vi "TEST-JSON-RPC.vi"() -> ()   [LabVIEW 2019, in "JSON-RPC.lvclass"]
uses:
  JSON-RPC.lvclass
  typedefs/Request--Cluster.ctl
  <vilib>/numeric/Random Number (Range) DBL.vi
  2af6048a-36b0-468c-b9d5-439df6bbc06a.vi
  423c0946-e876-4033-917c-c4e0f5a656b4.vi
  ba7f8204-1185-4351-9b6f-00361c30192e.vi
  2af6048a-36b0-468c-b9d5-439df6bbc06a.vi/56c0d29a-bd12-4556-9f6c-07d4d8114690.vi
  lv-venv/lv.lib/vi.lib/JDP Science/JSONtext/Make JSON Array.vi
  API/Create Batch Response.vi/8dac1c84-94f0-4a52-a653-2d1a946a353f.vi
  private/Parse Response-JSONtext.vi
  2af6048a-36b0-468c-b9d5-439df6bbc06a.vi/56c0d29a-bd12-4556-9f6c-07d4d8114690.vi/b1ff17d3-7a39-46cb-8eb5-aa197442e16a.vi
  API/Create Batch Response.vi/8dac1c84-94f0-4a52-a653-2d1a946a353f.vi/080af00f-872a-404d-81fb-91aec086d127.vi
  private/Parse Response-JSONtext.vi/7ce7fba8-9f44-478d-b6cb-b571ff29f2f5.vi
  private/Parse Response-JSONtext.vi/8c905beb-ab4c-49e3-b5c6-2c663b7b30d7.vi
  private/Parse Response-JSONtext.vi/fce5892e-0c40-47e1-88e0-6c122aadefe2.vi
  2af6048a-36b0-468c-b9d5-439df6bbc06a.vi/56c0d29a-bd12-4556-9f6c-07d4d8114690.vi/b1ff17d3-7a39-46cb-8eb5-aa197442e16a.vi/28d9b5f0-560b-4ba5-abe5-6e3ff87b2b6b.vi
  2af6048a-36b0-468c-b9d5-439df6bbc06a.vi/56c0d29a-bd12-4556-9f6c-07d4d8114690.vi/b1ff17d3-7a39-46cb-8eb5-aa197442e16a.vi/0d2768a8-5a07-4864-b3c8-f491049a930f.vi
  2af6048a-36b0-468c-b9d5-439df6bbc06a.vi/56c0d29a-bd12-4556-9f6c-07d4d8114690.vi/b1ff17d3-7a39-46cb-8eb5-aa197442e16a.vi/1e98635b-27c0-4b27-a2b5-38e38c963eb7.vi
  2af6048a-36b0-468c-b9d5-439df6bbc06a.vi/56c0d29a-bd12-4556-9f6c-07d4d8114690.vi/b1ff17d3-7a39-46cb-8eb5-aa197442e16a.vi/0d772b24-2de1-48ba-989a-96e16cd43241.vi
  2af6048a-36b0-468c-b9d5-439df6bbc06a.vi/56c0d29a-bd12-4556-9f6c-07d4d8114690.vi/b1ff17d3-7a39-46cb-8eb5-aa197442e16a.vi/3a44731f-0131-47ed-b9ac-c843c255cdb0.vi
  API/Create Batch Response.vi/8dac1c84-94f0-4a52-a653-2d1a946a353f.vi/080af00f-872a-404d-81fb-91aec086d127.vi/ddd97ab0-f880-4d62-a12b-adbfa2b80abd.vi
  API/Create Batch Response.vi/8dac1c84-94f0-4a52-a653-2d1a946a353f.vi/080af00f-872a-404d-81fb-91aec086d127.vi/db6e2d89-34ae-420f-86ba-38671ee62ba9.vi
  API/Create Batch Response.vi/8dac1c84-94f0-4a52-a653-2d1a946a353f.vi/080af00f-872a-404d-81fb-91aec086d127.vi/9674d577-b062-4377-a879-970cb02c3975.vi
  private/Create Error Object.vi
  lv-venv/lv.lib/vi.lib/JDP Science/JSONtext/Find Item.vi
  lv-venv/lv.lib/vi.lib/JDP Science/JSONtext/String Subset.vi
  <vilib>/Utility/Data Type/Get Type Information.vi
  lv-venv/lv.lib/vi.lib/JDP Science/JSONtext/Variant to JSON Text.vi
  lv-venv/lv.lib/vi.lib/JDP Science/JSONtext/Set Item.vi
  private/Create ID.vi
  lv-venv/lv.lib/vi.lib/JDP Science/JSONtext/support/Format JSON Array Text.vi
  lv-venv/lv.lib/vi.lib/JDP Science/JSONtext/JSON text to Variant.vi
  lv-venv/lv.lib/vi.lib/JDP Science/JSONtext/JSON type.vi
  lv-venv/lv.lib/vi.lib/JDP Science/JSONtext/Get Array Elements.vi
  lv-venv/lv.lib/vi.lib/JDP Science/JSONtext/Get all Object Items.vi
  lv-venv/lv.lib/vi.lib/JDP Science/JSONtext/Parsing/Parse Full Path or Item Name.vi
  lv-venv/lv.lib/vi.lib/JDP Science/JSONtext/Next JSON Value.vi
  lv-venv/lv.lib/vi.lib/JDP Science/JSONtext/support/Error Cluster From Code.vi
  lv-venv/lv.lib/vi.lib/JDP Science/JSONtext/Offset/Find Item Locations by Path.vi
  <vilib>/Utility/error.llb/Error Cluster From Error Code.vi
  lv-venv/lv.lib/vi.lib/JDP Science/JSONtext/LVClass Serializer/JSONtext LVClass Serializer.lvclass
panel:
  out "{JSON} Response":string
  out "{JSON} Requests":string
  out "error out":errorcluster
  out "4. parse response":dbl format="%#_6p"
  out "3. create response":dbl format="%#_6p"
  out "2. parse request":dbl format="%#_6p"
  out "1. create request":dbl format="%#_6p"
  out "Data out":dbl[](array[numeric])
  out "Params":string[](array[string])
  out "results":string[](array[string])
  out "Array":dbl[][](array[numeric])
  in  "Numeric":i32=3
  in  "Notification":bool
  in  "Request.method":string
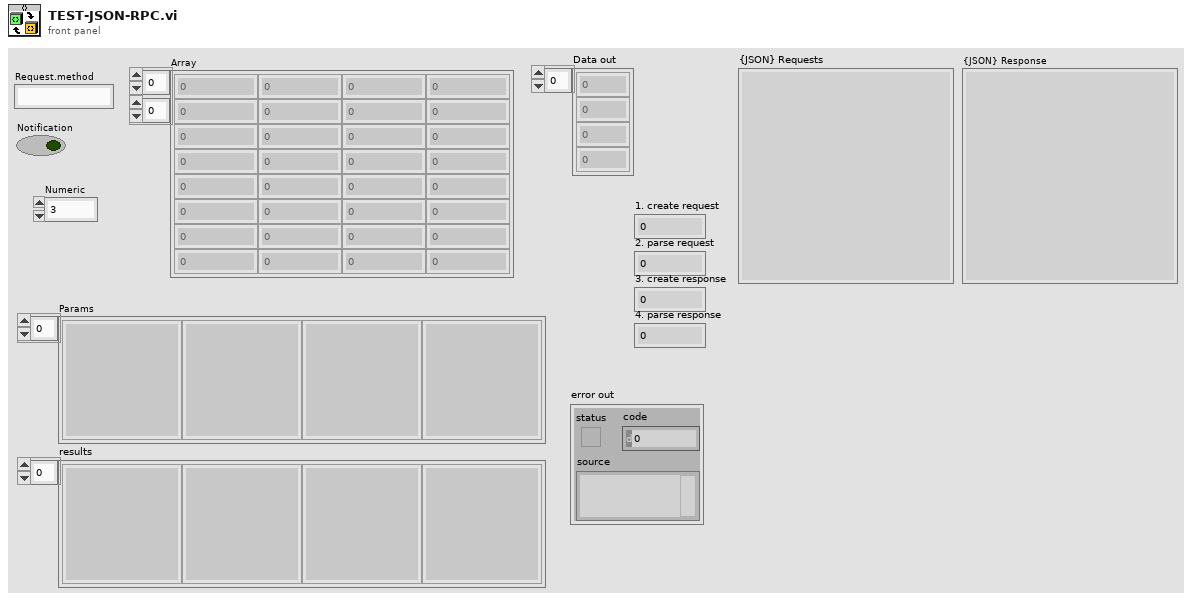
[diagram p1: front panel]
types:
  T1 = typedef "JSON-RPC.lvclass/Request--Cluster.ctl" = cluster{"method":string, "params":variant, "Notification?":bool}
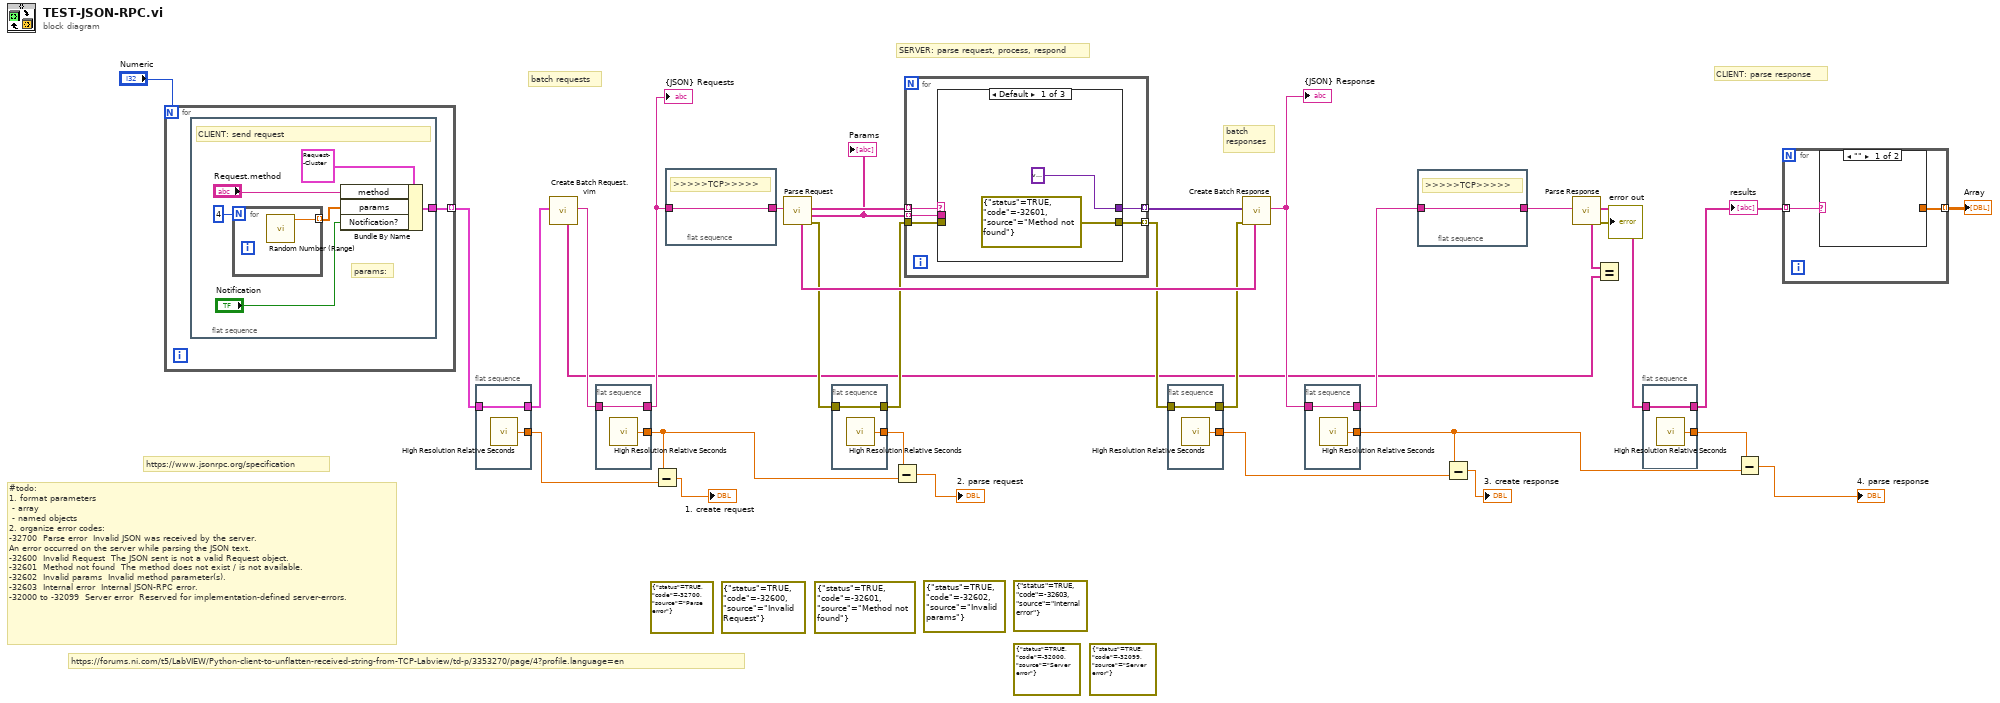
[diagram p0: block diagram]
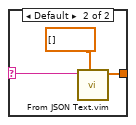
[diagram p2: hidden frame]
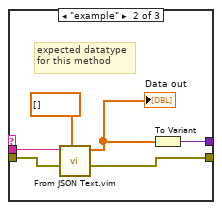
[diagram p3: hidden frame]
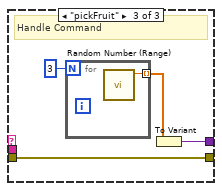
[diagram p4: hidden frame]
diagram:
  (unwired) errorcluster {"status"=TRUE, "code"=-32099, "source"="Server error"} ("error out")
  (unwired) errorcluster {"status"=TRUE, "code"=-32000, "source"="Server error"} ("error out")
  (unwired) errorcluster {"status"=TRUE, "code"=-32603, "source"="Internal error"} ("error out")
  (unwired) errorcluster {"status"=TRUE, "code"=-32601, "source"="Method not found"} ("error out")
  (unwired) errorcluster {"status"=TRUE, "code"=-32602, "source"="Invalid params"} ("error out")
  (unwired) errorcluster {"status"=TRUE, "code"=-32600, "source"="Invalid Request"} ("error out")
  (unwired) errorcluster {"status"=TRUE, "code"=-32700, "source"="Parse error"} ("error out")
  # "CLIENT: parse response"
  # "SERVER: parse request, process, respond"
  # "batch \nresponses"
  # "https://forums.ni.com/t5/LabVIEW/Python-client-to-unflatten-received-string-from-TCP-Labview/td-p/3353270/page/4?profile.language=en"
  # "#todo:\n1. format parameters\n - array\n - named objects\n2. organize error codes:\n-32700 \tParse error \tInvalid JSON was received by the server.\nAn error occurred on the server while parsing the JSON text.\n-32600 \tInvalid Request \tThe JSON sent is not a valid Request object.\n-32601 \tMethod not found \tThe method does not exist / is not available.\n-32602 \tInvalid params \tInvalid method parameter(s).\n-32603 \tInternal error \tInternal JSON-RPC error.\n-32000 to -32099 \tServer error \tReserved for implementation-defined server-errors."
  # "batch requests"
  # "https://www.jsonrpc.org/specification"
  n1 = for {
    N: "Numeric" -> [_]
    tunnel: [w34] -> w30 mode=indexing
    n2 = flat-sequence {
      tunnel: [w37] -> w34
      frame #0 {
        # "params:"
        # "CLIENT: send request"
        n3 = for {
          N: 4 -> [_]
          tunnel: [w41] -> w36 mode=indexing
          n4 = call-poly <vilib>:"Random Number (Range).vi"() -> ("number"=w41:dbl)  [unwired: 11 in]
        }
        n5 = Bundle By Name(cluster=T1 {"method"="", "params"=variant, "Notification?"=FALSE} ("request"), "method"="Request.method", "params"=w36, "Notification?"="Notification") -> (w37:T1)
      }
    }
  }
  n6 = flat-sequence {
    tunnel: [w42] -> w29
    tunnel: [w43] -> w28
    tunnel: w30 -> [w42]
    frame #0 {
      n7 = call <vilib>:"High Resolution Relative Seconds.vi"() -> ("relative seconds"=w43:dbl)
    }
  }
  n8 = call "Create Batch Request.vim"("Requests"=w29) -> ("{JSON} Requests"=w5:string, "ids"=w1:string[])  [unwired: 7 in, 2 out]
  n9 = flat-sequence {
    tunnel: [w44] -> w4
    tunnel: [w45] -> w21
    tunnel: w5 -> [w44]
    frame #0 {
      n10 = call <vilib>:"High Resolution Relative Seconds.vi"() -> ("relative seconds"=w45:dbl)
    }
  }
  n11 = Subtract(x=w21, y=w28) -> (x-y=→"1. create request":dbl)
  n12 = flat-sequence {
    tunnel: w4 -> [w46]
    tunnel: [w46] -> w3
    frame #0 {
      # ">>>>>TCP>>>>>"
    }
  }
  n13 = call "Parse Request.vi"("{JSON} Request"=w3) -> ("error out"=w23:errorcluster, "Params"=w26:string[], "Methods"=w27:string[], "ids"=w24:string[])  [unwired: 6 in, 1 out]
  "Params" <- w26
  n14 = flat-sequence {
    tunnel: [w47] -> w22
    tunnel: [w48] -> w17
    tunnel: w23 -> [w47]
    frame #0 {
      n15 = call <vilib>:"High Resolution Relative Seconds.vi"() -> ("relative seconds"=w48:dbl)
    }
  }
  n16 = Subtract(x=w17, y=w21) -> (x-y=→"2. parse request":dbl)
  n17 = for {
    tunnel: w26 -> [w52] mode=indexing
    tunnel: w27 -> [w51] mode=indexing
    tunnel: [w49] -> w25 mode=indexing
    tunnel: w22 -> [w53]
    tunnel: [w50] -> w19 mode=indexing
    n18 = case shown="Default" w51 {
      tunnel: w53 -> [_ w60 w65]
      tunnel: [errorcluster {"status"=TRUE, "code"=-32601, "source"="Method not found"} ("error out") w59 w65] -> w50
      tunnel: [variant ("Variant") w56 w63] -> w49
      tunnel: w52 -> [_ w61 _]
      frame Default {
      }
      frame "example" {
        # "expected datatype\nfor this method"
        n19 = call "From JSON Text.vim"("Data Type and Default Value"=dbl[] [], "error in (no error)"=w60, "JSON"=w61) -> ("error out"=w59:errorcluster, "Data out"=w57:dbl[])  [unwired: 7 in]
        "Data out" <- w57
        n20 = To Variant(anything=w57) -> (Variant=w56:variant)
      }
      frame "pickFruit" {
        # "Handle Command"
        n21 = for {
          N: 3 -> [_]
          tunnel: [w66] -> w62 mode=indexing
          n22 = call-poly <vilib>:"Random Number (Range).vi"() -> ("number"=w66:dbl)  [unwired: 11 in]
        }
        n23 = To Variant(anything=w62) -> (Variant=w63:variant)
      }
    }
  }
  n24 = flat-sequence {
    tunnel: [w67] -> w18
    tunnel: [w68] -> w13
    tunnel: w19 -> [w67]
    frame #0 {
      n25 = call <vilib>:"High Resolution Relative Seconds.vi"() -> ("relative seconds"=w68:dbl)
    }
  }
  n26 = call "Create Batch Response.vi"("ids"=w24, "error in (no error)"=w18, "results"=w25) -> ("{JSON} Response"=w15:string)  [unwired: 6 in, 2 out]
  "{JSON} Response" <- w15
  n27 = flat-sequence {
    tunnel: [w69] -> w14
    tunnel: [w70] -> w7
    tunnel: w15 -> [w69]
    frame #0 {
      n28 = call <vilib>:"High Resolution Relative Seconds.vi"() -> ("relative seconds"=w70:dbl)
    }
  }
  n29 = flat-sequence {
    tunnel: w14 -> [w71]
    tunnel: [w71] -> w33
    frame #0 {
      # ">>>>>TCP>>>>>"
    }
  }
  n30 = Subtract(x=w7, y=w13) -> (x-y=→"3. create response":dbl)
  n31 = call "Parse Response.vi"("{JSON} Response"=w33) -> ("error out"=→"error out":errorcluster, "results"=w10:string[], "ids"=w12:string[])  [unwired: 7 in, 1 out]
  n32 = Equal?(x=w12, y=w1) -> ()  [unwired: 1 out]
  n33 = flat-sequence {
    tunnel: [w72] -> w9
    tunnel: [w73] -> w8
    tunnel: w10 -> [w72]
    frame #0 {
      n34 = call <vilib>:"High Resolution Relative Seconds.vi"() -> ("relative seconds"=w73:dbl)
    }
  }
  n35 = Subtract(x=w8, y=w7) -> (x-y=→"4. parse response":dbl)
  n36 = for {
    tunnel: w9 -> [w74] mode=indexing
    tunnel: [w75] -> w11 mode=indexing
    n37 = case shown="\"\"" w74 {
      selector: w74 -> [_ w76]
      tunnel: [_ w77] -> w75
      frame "" {
      }
      frame Default {
        n38 = call "From JSON Text.vim"("Data Type and Default Value"=dbl[] [], "JSON"=w76) -> ("Data out"=w77:dbl[])  [unwired: 8 in, 1 out]
      }
    }
  }
  "Array" <- w11
  "results" <- w9
  "{JSON} Requests" <- w4
